vi "Greatest Common Divisor (GCD)-array input.vi"(8 "error in (no error)":errorcluster, 11 "Integers":i32[](array[numeric])) -> (0 "error out":errorcluster, 2 "T = x and y are relatively prime":bool, 3 "Greatest Common Divisor (GCD)":i32)   [LabVIEW 2021, in "Numeric Utilities.lvlib"]
uses:
  Numeric Utilities.lvlib
panel:
  out "Divisors that are common to all input integers":i32[](array[numeric])
  # "Development\ncontrols/indicators useful for development and testing, but which are not outputs of the VI"
  # "Input\nInputs to the VI"
  # "Output\nOutputs of the VI"
  # "Description\n\nBlank VI with error handling case. \n\nSummarize the use of this VI in this space."
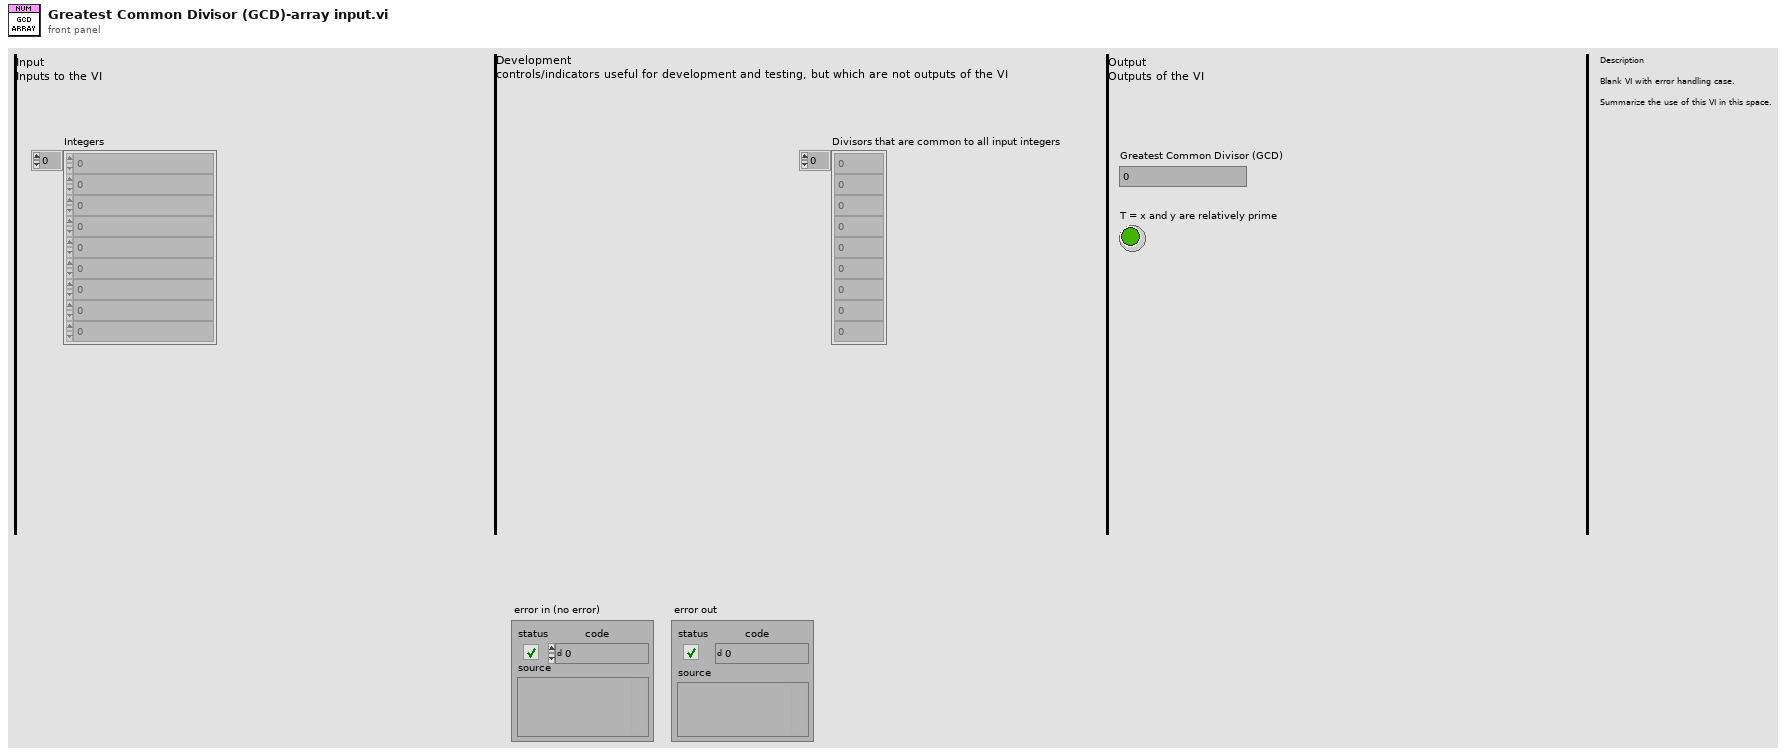
[diagram p1: front panel]
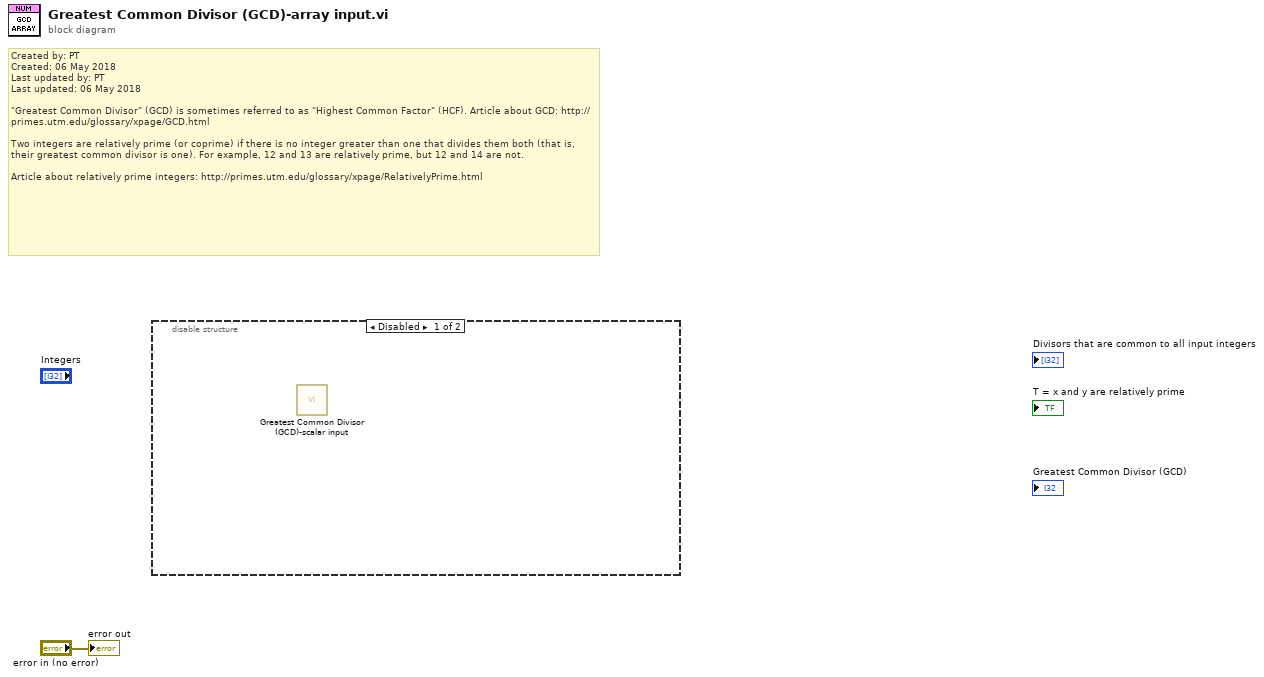
[diagram p0: block diagram]
diagram:
  # "Created by: PT\nCreated: 06 May 2018\nLast updated by: PT\nLast updated: 06 May 2018\n\n\"Greatest Common Divisor\" (GCD) is sometimes referred to as \"Highest Common Factor\" (HCF). Article about GCD: http://primes.utm.edu/glossary/xpage/GCD.html\n\nTwo integers are relatively prime (or coprime) if there is no integer greater than one that divides them both (that is, their greatest common divisor is one). For example, 12 and 13 are relatively prime, but 12 and 14 are not.\n\nArticle about relatively prime integers: http://primes.utm.edu/glossary/xpage/RelativelyPrime.html"
  n1 = disable-structure shown="Disabled" {
    frame Disabled {
      n2 = call "Greatest Common Divisor (GCD)-scalar input.vi"() -> ()  [unwired: 10 in, 2 out]
    }
    frame Enabled {
    }
  }
  "error out" <- "error in (no error)"
